vi "CR.vi"(8 "Sample Thickness (mm)":dbl, 9 "Sample Diameter (mm)":dbl, 10 "电压(V)":dbl, 11 "电流(A)":dbl) -> (1 "Resistivity (ohm·cm)":dbl, 2 "Current (A)":dbl, 3 "Resistance (ohm)":dbl)   [LabVIEW 2017]
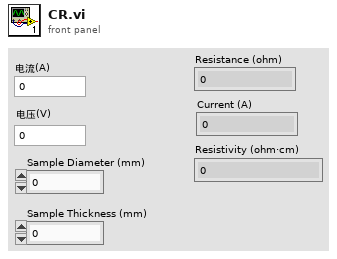
[diagram p1: front panel]
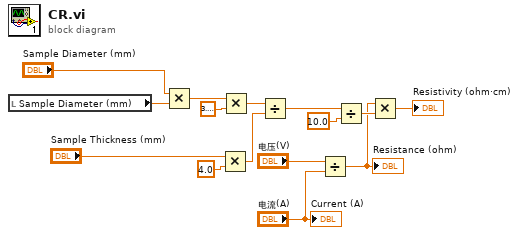
[diagram p0: block diagram]
diagram:
  n1 = local read "Sample Diameter (mm)"() -> (w14:dbl)
  n2 = Multiply(x="Sample Diameter (mm)", y=w14) -> (x*y=w13:dbl)
  n3 = Multiply(x="Sample Thickness (mm)", y=4.0) -> (x*y=w8:dbl)
  n4 = Multiply(x=w13, y=3.141592653589793) -> (x*y=w9:dbl)
  n5 = Divide(x=w9, y=w8) -> (x/y=w5:dbl)
  n6 = Divide(x="电压(V)", y="电流(A)") -> (x/y=w4:dbl)
  "Resistance (ohm)" <- w4
  n7 = Divide(x=w5, y=10.0) -> (x/y=w6:dbl)
  n8 = Multiply(x=w4, y=w6) -> (x*y=→"Resistivity (ohm·cm)":dbl)
  "Current (A)" <- "电流(A)"
